vi "measure-eventSD.vi"(1 "Controls":T1, 2 "error in":errorcluster, 3 "Cluster in":T2={"error"=refnum, "RT exp"=refnum, "# current"=refnum, "Start measurement"=refnum, "GRAPH EXPERIMENTAL DATA"=refnum, "DelaysTab"=enum."Table", "slider"=refnum, "aq contol"=enum."fixed", "RDT, ps"=refnum, "table delays"=[-500.0, -400.0, -0.0, 100.0, 250.0, 350.0], "notifier mesure in"=refnum, "Measure finished"=refnum, "Measure event"=refnum, "Laser shutter task"="", "minmaxOD"={"ODmin"=0.0, "ODmax"=0.0}}, 4 "Experiment in":refnum<class "Experiment.lvclass">, 5 "Operate":bool) -> (0 "error out":errorcluster)   [LabVIEW 2015]
uses:
  Classes/Experiment.lvclass
  controls/clustercontrols-measerument.ctl
  controls/Controls.ctl
  <vilib>/DAQmx/write.llb/DAQmx Write (Digital Bool 1Line 1Point).vi
  globalVarSD.vi
  <vilib>/DAQmx/miscellaneous.llb/DAQmx Fill In Error Info.vi
panel:
  in  "duration (msec)":u32=50 caption="durée (msec)"
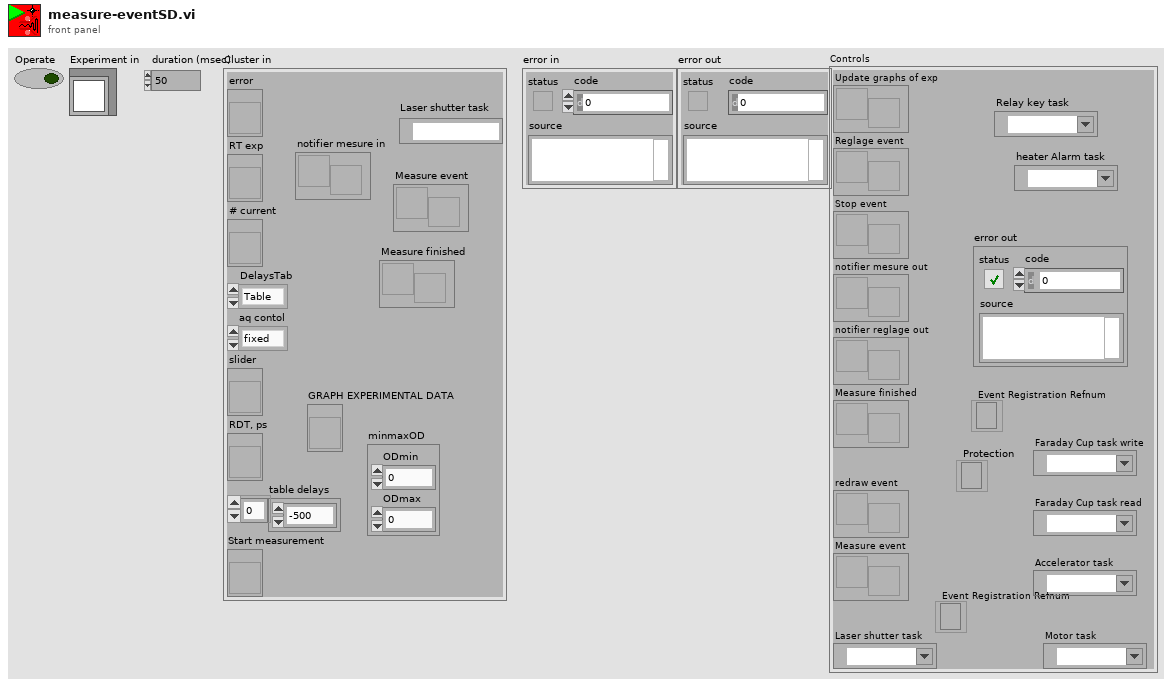
[diagram p1: front panel]
types:
  T1 = typedef "Controls.ctl" = cluster{"Update graphs of exp":refnum<user-event>, "Reglage event":refnum<user-event>, "Stop event":refnum<user-event>, "notifier mesure out":refnum<notifier>, "notifier reglage out":refnum<notifier>, "Measure finished":refnum<user-event>, "control registration ref":refnum<event-registration>, "redraw event":refnum<user-event>, "Measure event":refnum<user-event>, "Mes, Reg, Stop Registration ref":refnum<event-registration>, "Laser shutter task":refnum<k21>, "error out":errorcluster, "Motor task":refnum<k21>, "Accelerator task":refnum<k21>, "Faraday Cup task read":refnum<k21>, "Protection":refnum<event-registration>, "heater Alarm task":refnum<k21>, "Relay key task":refnum<k21>, "Faraday Cup task write":refnum<k21>}
  T2 = typedef "clustercontrols-measerument.ctl" = cluster{"error":refnum<vi>, "RT exp":refnum<vi>, "# current":refnum<vi>, "Start measurement":refnum<vi>, "GRAPH EXPERIMENTAL DATA":refnum<vi>, "DelaysTab":enum32{"Mode Normale", "Table"}, "slider":refnum<vi>, "aq contol":enum32{"fixed", "automatic", "fixed-auto"}, "RDT, ps":refnum<vi>, "table delays":dbl[], "notifier mesure in":refnum<notifier>, "Measure finished":refnum<user-event>, "Measure event":refnum<user-event>, "Laser shutter task":refnum<k21>, "minmaxOD":cluster{"ODmin":dbl, "ODmax":dbl}}
  T3 = cluster{"Operate":bool, "Experiment out":refnum<class "Experiment.lvclass">}
  T4 = cluster{"Operate":bool, "Experiment out":refnum<class "Experiment.lvclass">, path}
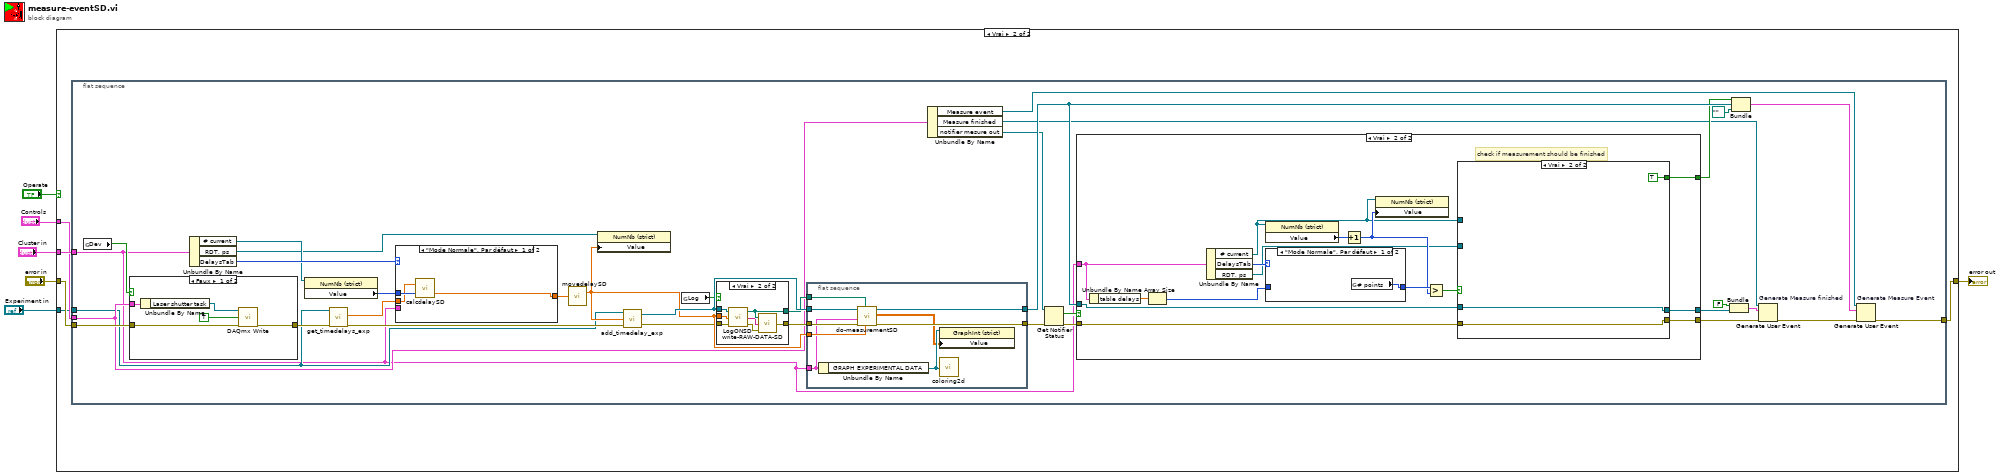
[diagram p0: block diagram]
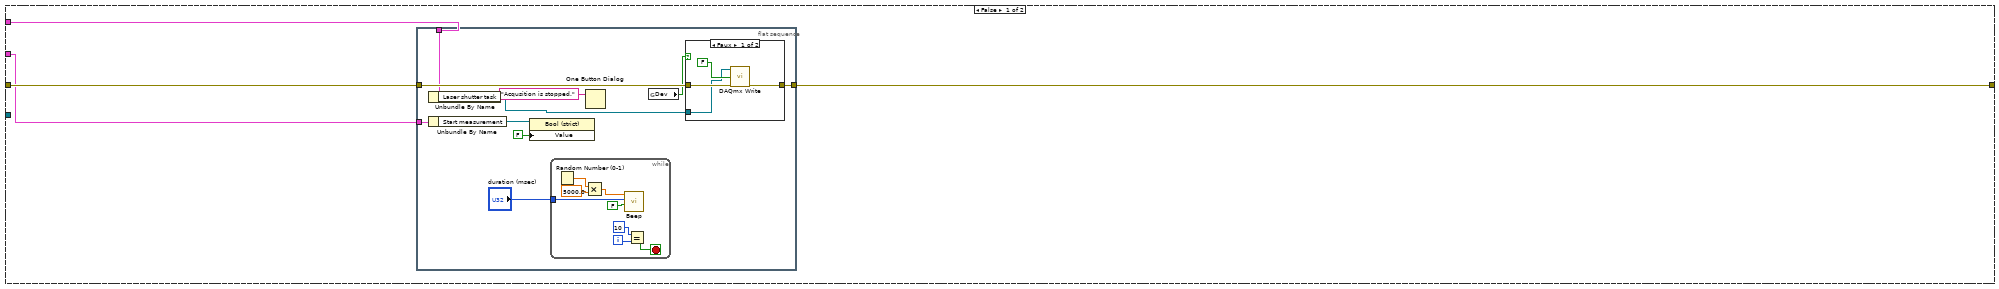
[diagram p2: hidden frame]
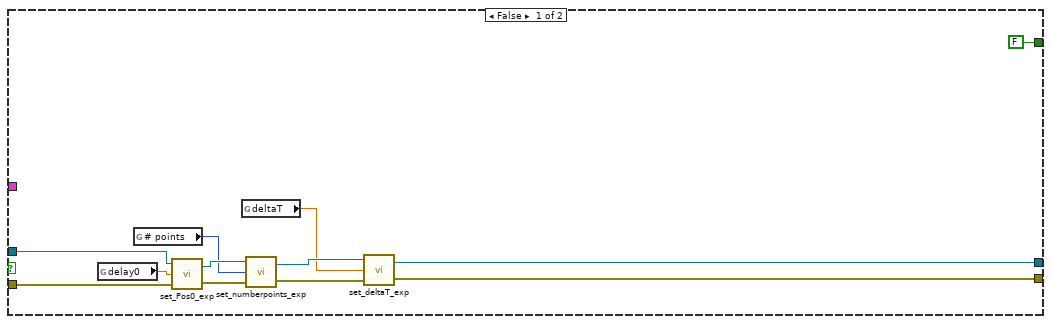
[diagram p4: hidden frame]
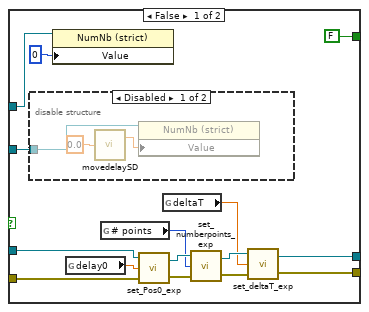
[diagram p6: hidden frame]
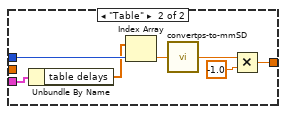
[diagram p9: hidden frame]
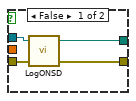
[diagram p10: hidden frame]
diagram:
  n1 = case shown="Vrai" "Operate" {
    tunnel: "error in" -> [w10 w36]
    tunnel: [w9 w38] -> w6
    tunnel: "Cluster in" -> [w8 w37]
    tunnel: "Controls" -> [w7 w35]
    tunnel: "Experiment in" -> [_ w34]
    frame False {
      n2 = flat-sequence {
        tunnel: w10 -> [w17]
        tunnel: [w16] -> w9
        tunnel: w8 -> [w14]
        tunnel: w7 -> [w12]
        frame #0 {
          n3 = Unbundle By Name(w12) -> ("Laser shutter task"=w11:refnum<k21>)
          n4 = Unbundle By Name(w14) -> ("Start measurement"=w13:refnum<vi>)
          n5 = property class="Bool (strict)"(reference=w13, "Value"=FALSE) -> ()  [unwired: 1 in, 2 out]
          n6 = while {
            tunnel: "duration (msec)" -> [w29]
            i -> [w28]
            stop <- w26 stop-if-true
            n7 = Random Number (0-1)() -> (number: 0 to 1=w32:dbl)
            n8 = Multiply(x=w32, y=5000.0) -> (x*y=w30:dbl)
            n9 = call <vilib>:"Beep.vi"("use system alert? (T)"=FALSE, "duration (msec)"=w29, "frequency (Hz)"=w30) -> ()  [unwired: 9 in]
            n10 = Equal?(x=10, y=w28) -> (x = y?=w26:bool)
          }
          n11 = One Button Dialog(message="Acqusition is stopped.") -> ()  [unwired: 1 in, 1 out]
          n12 = global read "globalVarSD.vi" "Dev"() -> (w15:bool)
          n13 = case shown="Faux" w15 {
            tunnel: w17 -> [w23 w25]
            tunnel: [w22 w25] -> w16
            tunnel: w11 -> [w21 _]
            frame False {
              n14 = call-poly <vilib>:"DAQmx Write.vi"("task/channels in"=w21, "data"=FALSE, "error in"=w23) -> ("error out"=w22:errorcluster)  [unwired: 10 in, 2 out]
            }
            frame True {
            }
          }
        }
      }
    }
    frame True {
      n15 = flat-sequence {
        tunnel: [w73] -> w38
        tunnel: w37 -> [w39]
        tunnel: w36 -> [w70]
        tunnel: w35 -> [w41]
        tunnel: w34 -> [w40]
        frame #0 {
          n16 = global read "globalVarSD.vi" "Dev"() -> (w60:bool)
          n17 = case shown="Faux" w60 {
            tunnel: w70 -> [w137 w138]
            tunnel: [w136 w138] -> w56
            tunnel: w41 -> [w133 _]
            frame False {
              n18 = Unbundle By Name(w133) -> ("Laser shutter task"=w134:refnum<k21>)
              n19 = call-poly <vilib>:"DAQmx Write.vi"("task/channels in"=w134, "data"=TRUE, "error in"=w137) -> ("error out"=w136:errorcluster)  [unwired: 10 in, 2 out]
            }
            frame True {
            }
          }
          n20 = Unbundle By Name(w39) -> ("# current"=w58:refnum<vi>, "RDT, ps"=w57:refnum<vi>, "DelaysTab"=w59:enum32{"Mode Normale", "Table"})
          n21 = property class="NumNb (strict)"(reference=w58) -> ("Value"=w65:i32)  [unwired: 1 in, 2 out]
          n22 = call-dynamic "get_timedelays_exp.vi"("error in (no error)"=w56, "Experiment.lvclass in"=w40) -> ("error out"=w55:errorcluster, "timedelays"=w61:dbl[])  [unwired: 7 in, 1 out]
          n23 = case shown="\"Mode Normale\", Par défaut" w59 {
            tunnel: w65 -> [w141 w148]
            tunnel: [w140 w144] -> w64
            tunnel: w61 -> [w139 _]
            tunnel: w39 -> [_ w142]
            frame "Mode Normale", Default {
              n24 = call "calcdelaySD.vi"("current point"=w141, "timedelays"=w139) -> ("Delay, mm"=w140:dbl)  [unwired: 1 in]
            }
            frame "Table" {
              n25 = Unbundle By Name(w142) -> ("table delays"=w143:dbl[])
              n26 = Index Array(array=w143, index=w148) -> (element=w145:dbl)
              n27 = call "convertps-to-mmSD.vi"("ps"=w145) -> ("mm"=w146:dbl)
              n28 = Multiply(x=w146, y=-1.0) -> (x*y=w144:dbl)
            }
          }
          n29 = call "movedelaySD.vi"("Delay, mm"=w64) -> ("Real delay time, ps"=w67:dbl)  [unwired: 1 out]
          n30 = property class="NumNb (strict)"(reference=w57, "Value"=w67) -> ()  [unwired: 1 in, 2 out]
          n31 = call-dynamic "add_timedelay_exp.vi"("error in (no error)"=w55, "delay"=w67, "Experiment.lvclass in"=w40) -> ("error out"=w62:errorcluster, "Experiment.lvclass out"=w69:refnum<class "Experiment.lvclass">)
          n32 = global read "globalVarSD.vi" "Log"() -> (w63:bool)
          n33 = case shown="Vrai" w63 {
            tunnel: w62 -> [w150 w159]
            tunnel: [w151 w158] -> w66
            tunnel: w69 -> [w152 w157]
            tunnel: [w149 w153] -> w68
            tunnel: w67 -> [_ w156]
            frame False {
              n34 = call "LogONSD.vi"("error in (no error)"=w150, "Experiment in"=w152) -> ("error out"=w149:errorcluster, "Path"=w151:path)  [unwired: 1 in, 1 out]
            }
            frame True {
              n35 = call "LogONSD.vi"("error in (no error)"=w159, "Real delay time, ps"=w156, "Experiment in"=w157) -> ("error out"=w154:errorcluster, "String"=w155:string, "Path"=w158:path)
              n36 = call "write-RAW-DATA-SD.vi"("error in (no error)"=w154, "Text"=w155, "File"=w158) -> ("error out"=w153:errorcluster)
            }
          }
          n37 = flat-sequence {
            tunnel: [w82] -> w72
            tunnel: [w81] -> w71
            tunnel: w69 -> [w80]
            tunnel: w68 -> [w79]
            tunnel: w67 -> [w78]
            tunnel: w66 -> [w77]
            tunnel: w39 -> [w75]
            frame #0 {
              n38 = Unbundle By Name(w75) -> ("GRAPH EXPERIMENTAL DATA"=w76:refnum<vi>)
              n39 = call "do-measurementSD.vi"("Real delay time, ps"=w78, "File"=w77, "error in (no error)"=w79, "Cluster in"=w75, "Experiment in"=w80) -> ("error out"=w82:errorcluster, "graph data"=w74:dbl[][], "Experiment out"=w81:refnum<class "Experiment.lvclass">)  [unwired: 4 in]
              n40 = property class="GraphInt (strict)"(reference=w76, "Value"=w74) -> ()  [unwired: 1 in, 2 out]
              n41 = call "coloring2d.vi"("reference graph"=w76) -> ()  [unwired: 1 in]
            }
          }
          n42 = Unbundle By Name(w41) -> ("Measure event"=w45:refnum<user-event>, "Measure finished"=w46:refnum<user-event>, "notifier mesure out"=w47:refnum<notifier>)
          n43 = Get Notifier Status(notifier=w47, error in (no error)=w72) -> (current notification=w54:bool, error out=w42:errorcluster)  [unwired: 3 out]
          n44 = case shown="Vrai" w54 {
            tunnel: [FALSE ("Operate") w108] -> w53
            tunnel: w71 -> [w89 w107]
            tunnel: [w88 w105] -> w48
            tunnel: w39 -> [_ w96]
            tunnel: w42 -> [w84 w99]
            tunnel: [w83 w98] -> w44
            frame False {
              n45 = global read "globalVarSD.vi" "delay0"() -> (w87:dbl)
              n46 = global read "globalVarSD.vi" "# points"() -> (w85:i32)
              n47 = call-dynamic "set_Pos0_exp.vi"("error in (no error)"=w84, "Pos0,ps"=w87, "Experiment.lvclass in"=w89) -> ("error out"=w91:errorcluster, "Experiment.lvclass out"=w92:refnum<class "Experiment.lvclass">)
              n48 = global read "globalVarSD.vi" "deltaT"() -> (w86:dbl)
              n49 = call-dynamic "set_numberpoints_exp.vi"("error in (no error)"=w91, "numberpoints"=w85, "Experiment.lvclass in"=w92) -> ("error out"=w90:errorcluster, "Experiment.lvclass out"=w93:refnum<class "Experiment.lvclass">)
              n50 = call-dynamic "set_deltaT_exp.vi"("error in (no error)"=w90, "deltaTlast"=w86, "Experiment.lvclass in"=w93) -> ("error out"=w83:errorcluster, "Experiment.lvclass out"=w88:refnum<class "Experiment.lvclass">)
            }
            frame True {
              # "check if measurement should be finished"
              n51 = Unbundle By Name(w96) -> ("table delays"=w97:dbl[])
              n52 = Array Size(array=w97) -> (size(s)=w95:i32)
              n53 = Unbundle By Name(w96) -> ("# current"=w102:refnum<vi>, "DelaysTab"=w101:enum32{"Mode Normale", "Table"}, "RDT, ps"=w100:refnum<vi>)
              n54 = property class="NumNb (strict)"(reference=w102) -> ("Value"=w106:i32)  [unwired: 1 in, 2 out]
              n55 = case shown="\"Mode Normale\", Par défaut" w101 {
                tunnel: [w110 w111] -> w104
                tunnel: w95 -> [_ w111]
                frame "Mode Normale", Default {
                  n56 = global read "globalVarSD.vi" "# points"() -> (w110:i32)
                }
                frame "Table" {
                }
              }
              n57 = Increment(x=w106) -> (x+1=w103:i32)
              n58 = property class="NumNb (strict)"(reference=w102, "Value"=w103) -> ()  [unwired: 1 in, 2 out]
              n59 = Greater?(x=w104, y=w103) -> (0:w109:bool)
              n60 = case shown="Vrai" w109 {
                tunnel: w107 -> [w117 w131]
                tunnel: [FALSE ("Operate") TRUE ("Operate")] -> w108
                tunnel: w100 -> [w125 _]
                tunnel: w102 -> [w123 _]
                tunnel: [w114 w131] -> w105
                tunnel: w99 -> [w113 w130]
                tunnel: [w112 w130] -> w98
                frame False {
                  n61 = disable-structure shown="Disabled" {
                    disable-tunnel: w125 -> [w127 _]
                    frame Disabled {
                      n62 = call "movedelaySD.vi"("Delay, mm"=0.0) -> ("Real delay time, ps"=w129:dbl)  [unwired: 1 out]
                      n63 = property class="NumNb (strict)"(reference=w127, "Value"=w129) -> ()  [unwired: 1 in, 2 out]
                    }
                    frame Enabled {
                    }
                  }
                  n64 = property class="NumNb (strict)"(reference=w123, "Value"=0 ("Nombre de point indic")) -> ()  [unwired: 1 in, 2 out]
                  n65 = global read "globalVarSD.vi" "delay0"() -> (w116:dbl)
                  n66 = global read "globalVarSD.vi" "# points"() -> (w115:i32)
                  n67 = call-dynamic "set_Pos0_exp.vi"("error in (no error)"=w113, "Pos0,ps"=w116, "Experiment.lvclass in"=w117) -> ("error out"=w120:errorcluster, "Experiment.lvclass out"=w121:refnum<class "Experiment.lvclass">)
                  n68 = global read "globalVarSD.vi" "deltaT"() -> (w118:dbl)
                  n69 = call-dynamic "set_numberpoints_exp.vi"("error in (no error)"=w120, "numberpoints"=w115, "Experiment.lvclass in"=w121) -> ("error out"=w119:errorcluster, "Experiment.lvclass out"=w122:refnum<class "Experiment.lvclass">)
                  n70 = call-dynamic "set_deltaT_exp.vi"("error in (no error)"=w119, "deltaTlast"=w118, "Experiment.lvclass in"=w122) -> ("error out"=w112:errorcluster, "Experiment.lvclass out"=w114:refnum<class "Experiment.lvclass">)
                }
                frame True {
                }
              }
            }
          }
          n71 = Bundle("Operate"=FALSE, "Experiment out"=w48) -> (w50:T3)  [unwired: 1 in]
          n72 = Bundle("Operate"=w53, "Experiment out"=w71, path "") -> (w52:T4)  [unwired: 1 in]
          n73 = Generate User Event "Generate Measure finished"(user event=w46, event data cluster=w50, error in=w44) -> (error out=w43:errorcluster)  [unwired: 1 in, 1 out]
          n74 = Generate User Event "Generate Measure Event"(user event=w45, event data cluster=w52, error in=w43) -> (error out=w73:errorcluster)  [unwired: 1 in, 1 out]
        }
      }
    }
  }
  "error out" <- w6
